vi "4.vi"(8 "Error In":errorcluster, 11 "buffer in":cluster{"PIPE IN":i32, "PIPE OUT":i32}) -> (0 "Error Out":errorcluster, 3 "cierre":bool)   [LabVIEW 2016]
uses:
  microchip_solutions_v2013-06-15/USB/Tools/MCHPUSB Custom Driver/Mpusbapi/Dll/Borland_C/Source/mpusbapi.dll
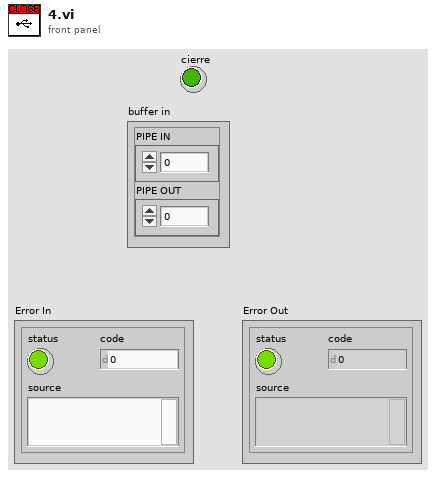
[diagram p1: front panel]
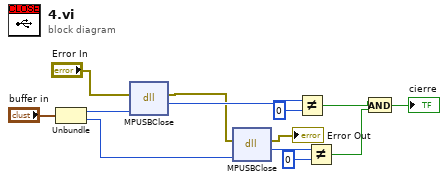
[diagram p0: block diagram]
diagram:
  n1 = Unbundle("buffer in") -> ("PIPE IN"=w6:i32, "PIPE OUT"=w5:i32)
  n2 = dll-call lib="C:/microchip_solutions_v2013-06-15/USB/Tools/MCHPUSB Custom Driver/Mpusbapi/Dll/Borland_C/Source/mpusbapi.dll" fn="MPUSBClose"(error in="Error In", "PIPE"=w6) -> (error out=w2:errorcluster, "BOOL"=w13:i32)  [unwired: 3 in, 1 out]
  n3 = dll-call lib="C:/microchip_solutions_v2013-06-15/USB/Tools/MCHPUSB Custom Driver/Mpusbapi/Dll/Borland_C/Source/mpusbapi.dll" fn="MPUSBClose"(error in=w2, "PIPE"=w5) -> (error out=→"Error Out":errorcluster, "BOOL"=w9:i32)  [unwired: 3 in, 1 out]
  n4 = Not Equal?(x=w13, y=0) -> (x != y?=w8:bool)
  n5 = Not Equal?(x=w9, y=0) -> (x != y?=w3:bool)
  n6 = And(x=w8, y=w3) -> (x .and. y?=→"cierre":bool)
